vi "Delete AO Endpoint.vi"(0 "Tosca in":refnum<class "Parameters.lvclass">, 7 "FSM.Graph":refnum<class "FSM.Graph.lvclass">, 9 "Old name":string, 11 "error in (no error)":errorcluster) -> (4 "Tosca out":refnum<class "Parameters.lvclass">, 8 "FSM.Graph Out":refnum<class "FSM.Graph.lvclass">, 15 "error out":errorcluster)   [LabVIEW 2020, in "Parameters.lvclass"]
uses:
  Parameters.lvclass
  FSM Graph VIs/LV Source/Classes/FSM.Graph/FSM.Graph.lvclass
  Parameters.lvclass/Parameters.ctl
  FSM Graph VIs/LV Source/Classes/FSM.Node/Badge.ctl
  State/State.lvclass/State.ctl
  State/Read SigMan.vi
  State/Write SigMan.vi
  epl-vi-lib/Signal Synthesis VIs/4th Generation/Classes/SignalManager/SignalManager.lvclass
  State/State.lvclass
  FSM Graph VIs/LV Source/Classes/FSM.Node/FSM.Node.lvclass
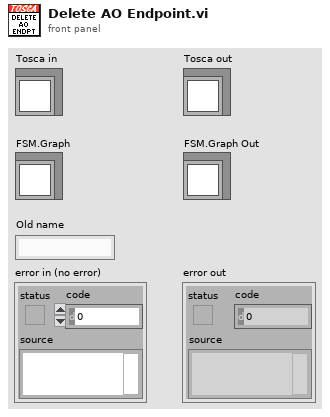
[diagram p1: front panel]
types:
  T1 = typedef "FSM.Node.lvclass/Badge.ctl" = enum16{"Audio", "Visual"}
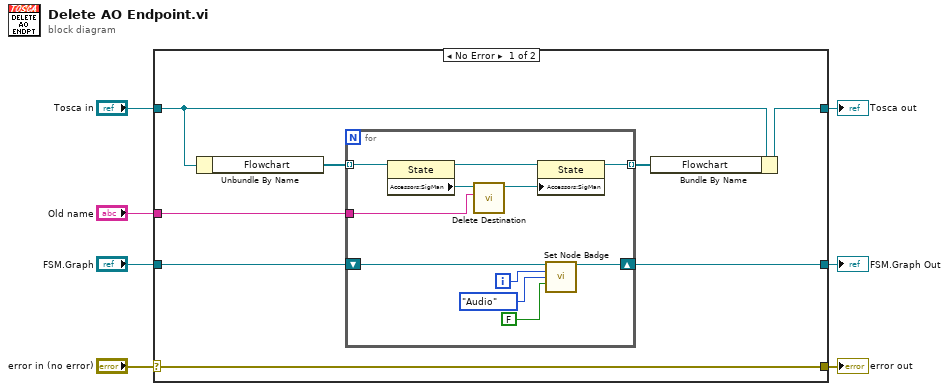
[diagram p0: block diagram]
diagram:
  n1 = case shown="No Error" "error in (no error)" {
    selector: "error in (no error)" -> [w15 w29]
    tunnel: [w15 w29] -> w6
    tunnel: [w12 w28] -> w4
    tunnel: "Tosca in" -> [w14 w28]
    tunnel: "Old name" -> [w10 _]
    tunnel: [w8 w27] -> w2
    tunnel: "FSM.Graph" -> [w9 w27]
    frame No Error {
      n2 = Unbundle By Name(w14) -> ("Flowchart"=w13:refnum<class "State.lvclass">[])
      n3 = for {
        tunnel: w13 -> [w26] mode=indexing
        tunnel: [w22] -> w11 mode=indexing
        tunnel: w10 -> [w21]
        shift-right: [w19] -> w8
        shift-left: w9 -> [w20]
        i -> [w18]
        n4 = property class="State"(reference=w26) -> (reference out=w24:refnum<class "State.lvclass">, "Accessors:SigMan"=w25:refnum<class "SignalManager.lvclass">)  [unwired: 1 in, 1 out]
        n5 = call "Delete Destination.vi"("Name"=w21, "SigMan in"=w25) -> ("SigMan out"=w23:refnum<class "SignalManager.lvclass">)  [unwired: 8 in, 1 out]
        n6 = property class="State"(reference=w24, "Accessors:SigMan"=w23) -> (reference out=w22:refnum<class "State.lvclass">)  [unwired: 1 in, 1 out]
        n7 = call "Set Node Badge.vi"("FSM in"=w20, "nodeIndex"=w18, "Badge"=Badge."Audio", "visible"=FALSE) -> ("FSM out"=w19:refnum<class "FSM.Graph.lvclass">)  [unwired: 10 in, 1 out]
      }
      n8 = Bundle By Name(cluster=w14, "Flowchart"=w11) -> (w12:refnum<class "Parameters.lvclass">)
    }
    frame Error {
    }
  }
  "error out" <- w6
  "Tosca out" <- w4
  "FSM.Graph Out" <- w2
